vi "PH_SHS_Analysis_Calibrator.panel.vi"(0 "object ref":refnum<vi>, 5 "error in (no error)":errorcluster) -> (19 "error out":errorcluster)   [LabVIEW 2014, in "PH_SHS_Analysis_Calibrator.lvlib"]
doc: "The voltage measured by a device on high potential is represented by a frequency given out by a Beckhoff Klemme. This VI transforms it back into a voltage which wich is written to a memory tag. This value is indicated. In case of no connection (not mounted or bad tag value) or internal problems \"99999\" apears.\n\n\"Exit\" closes the GUI while \"Delete Instance\" additionally destroys the Instance.\n\n\n\nLicense Agreement for this software:\n\nCopyright (C)\nGesellschaft für Schwerionenforschung, GSI\nPlanckstr. 1\n64291 Darmstadt\nGermany\n\nContact: D.Beck@gsi.de \n\nThis program is free software; you can redistribute it and/or modify it under the terms of the GNU General Public License as published by the Free Software Foundation; either version 2 of the license, or (at your option) any later version.\n\nThis program is distributed in the hope that it will be useful, but WITHOUT ANYW ARRANTY; without even the implied warranty of MERCHANTABILITY or FITNESS FOR A PARTICULAR PURPOSE. See the GNU General License for more details (http://www.gnu.org).\n\nGesellschaft für Schwerionenforschung, GSI\nPlanckstr. 1, 64291 Darmstadt, Germany\nFor all questions and ideas contact: M.Richter@gsi.de, H.Brand@gsi.de or D.Beck@gsi.de.\nLast update: 18-DEC-2002"
uses:
  PH_SHS_Analysis_Calibrator.lvlib
  PH_Img_BaseClass/PH_Img_BaseClass.Palette.ctl
  PH_Img_BaseClass/PH_Img_BaseClass.GUI Refs.ctl
  PH_Common/PH_Common.lvlib
  PH_Img_BaseClass/PH_Img_BaseClass.lvlib
  CSCore/CSSystem/CSSystemLib/CSSystemLib.lvlib
  PH_Class/PH_Class.lvlib
panel:
  in  "Timeout Set":i32 caption="ms"
  in  "Palette":T1 items=["Grey", "Binary", "Gradient", "Rainbow", "Temperature"]
  out "Timeout":u32(colorbox)=16860
  out "Enough Images?":bool
  in  "Method":enum16{"automatic", "manual"}(ring)
  in  "MLA Pitch":dbl=200.0 caption="µm"
  in  "Pixel Size":dbl=6.7 caption="µm"
  out "Image":T2(plugin-control)
  out "Dialog":string
  in  "Repeat":bool
  in  "Skip":bool
  in  "Cancel":bool
  in  "OK":bool
  in  "Available Cams":u16(ring)
  in  "Delete":bool
  # "PCS"
  # "3.40"
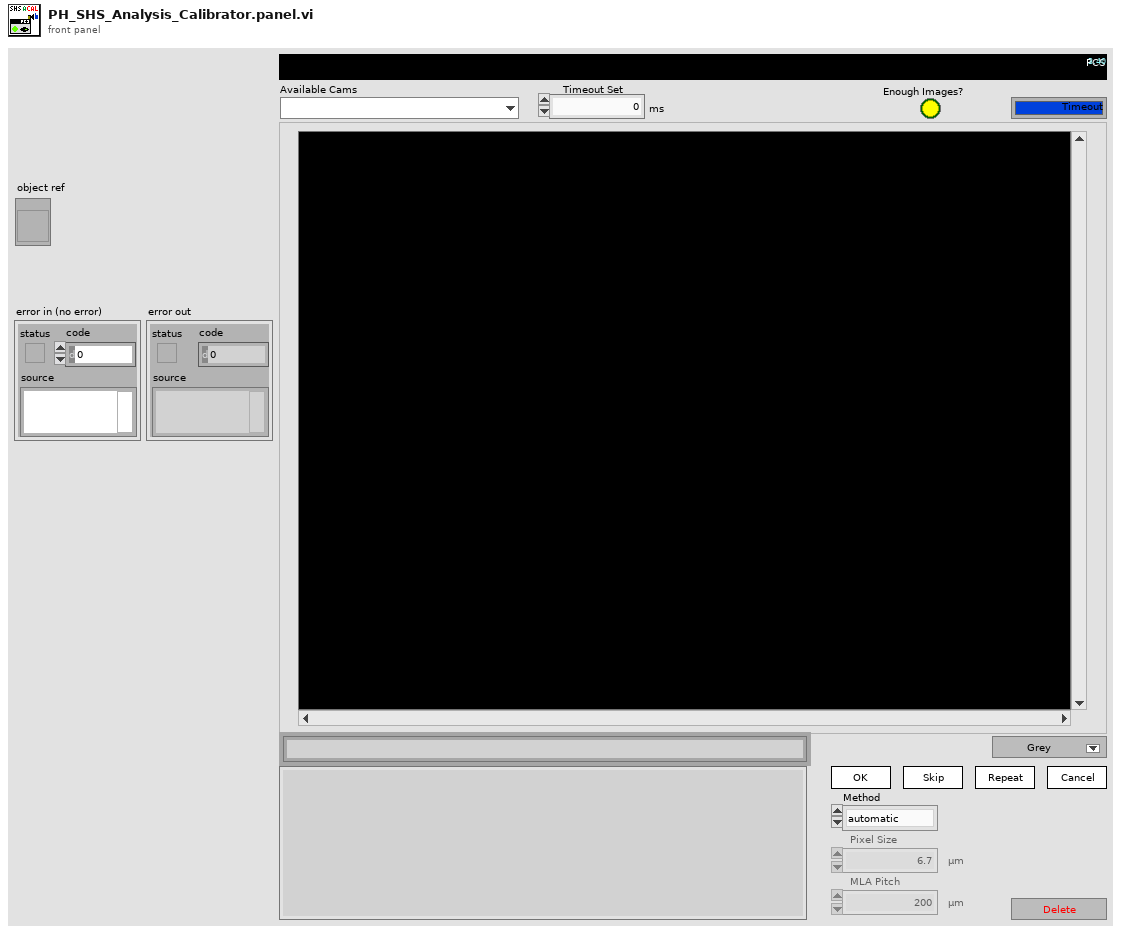
[diagram p1: front panel]
types:
  T1 = typedef "PH_Img_BaseClass.lvlib/PH_Img_BaseClass.Palette.ctl" = i32
  T2 = typedef "IMAQ Image.ctl" = refnum<image>
  T3 = typedef "PH_Img_BaseClass.lvlib/PH_Img_BaseClass.GUI Refs.ctl" = cluster{"Timeout":refnum<vi>, "Image":refnum<vi>, "Palette":refnum<vi>, "Timeout Set":refnum<vi>}
  T4 = enum8{"Enabled", "Disabled", "Disabled and Grayed Out"}
  T5 = typedef "PH_SHS_Analysis_Calibrator.lvlib/PH_SHS_Analysis_Calibrator.i attribute.ctl" = cluster{"GUI Refs":cluster{"Available Cams":refnum<vi>, "OK":refnum<vi>, "Skip":refnum<vi>, "Repeat":refnum<vi>, "Cancel":refnum<vi>, "Dialog":refnum<vi>, "Enough Images?":refnum<vi>}, "Cam instances":string[], "Status":cluster{"#":i32, "Data calculated":bool, "Wanted #":i32}, "IMAQ Image Array":T2[], "Pixel Size [µm]":dbl, "MLA Pitch [µm]":dbl, "Method":enum16{"automatic", "manual"}, "Enough Images?":bool, "SHS Reference Result":T6, "Calculation Error":errorcluster}
  T6 = typedef "SHS_Common.lvlib/SHSReference.ctl" = cluster{"Reference":T7[][], "Lens Array Pitch [px]":dbl}
  T7 = typedef "SHS_Common.lvlib/ReferencePoint.ctl" = cluster{"Rect":T8, "Point":T9}
  T8 = typedef "SHS_Common.lvlib/Rectangle.ctl" = cluster{"Left":i32, "Top":i32, "Right":i32, "Bottom":i32}
  T9 = typedef "SHS_Common.lvlib/Point.ctl" = cluster{"x":dbl, "y":dbl, "valid?":bool, "weight":dbl}
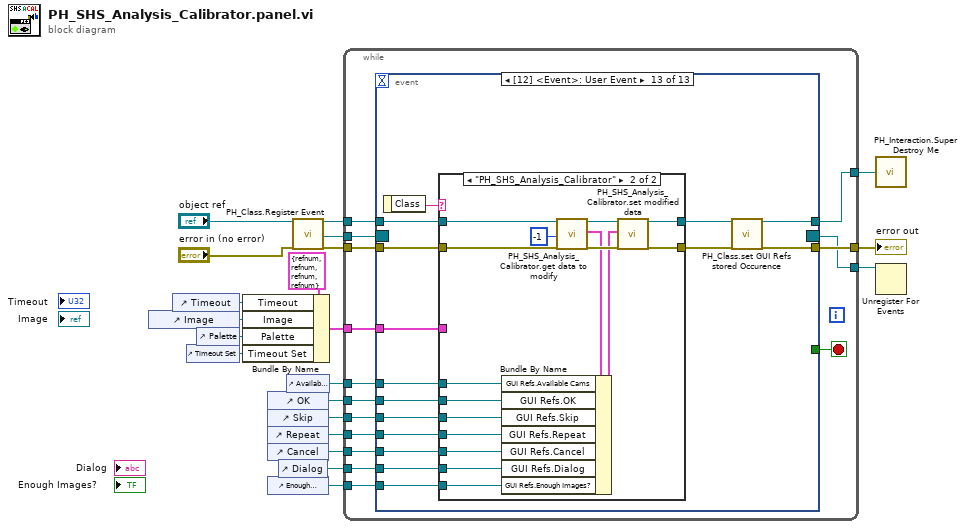
[diagram p0: block diagram]
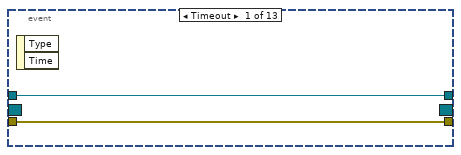
[diagram p2: hidden frame]
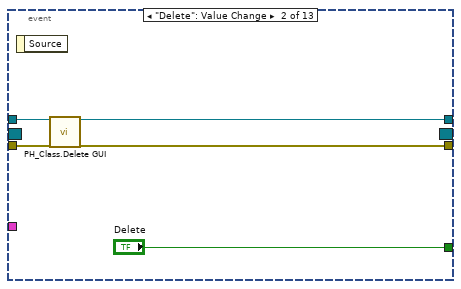
[diagram p3: hidden frame]
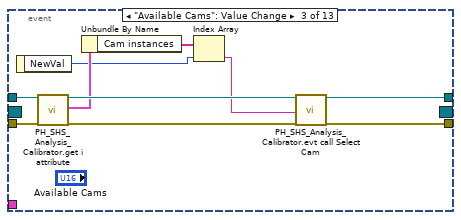
[diagram p4: hidden frame]
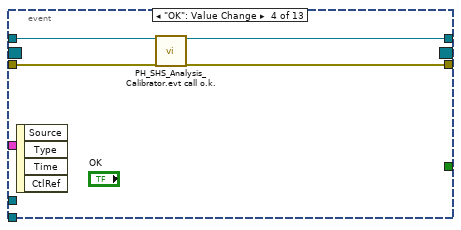
[diagram p5: hidden frame]
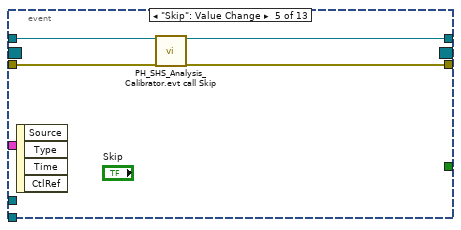
[diagram p6: hidden frame]
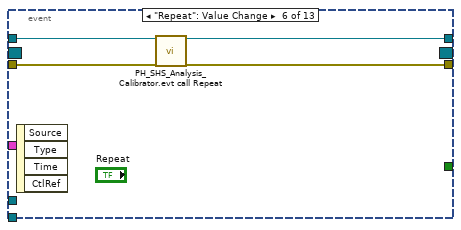
[diagram p7: hidden frame]
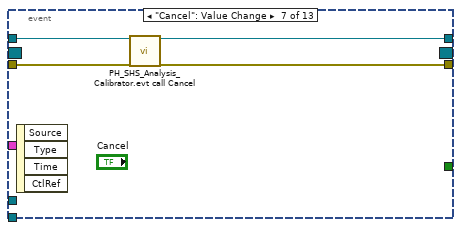
[diagram p8: hidden frame]
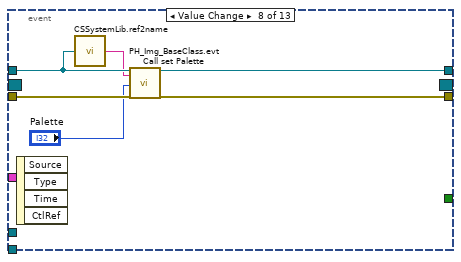
[diagram p9: hidden frame]
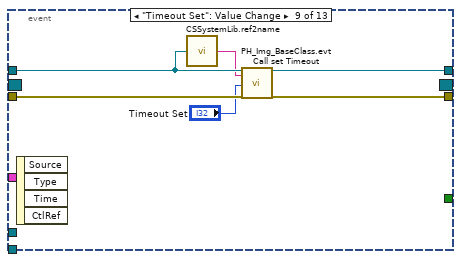
[diagram p10: hidden frame]
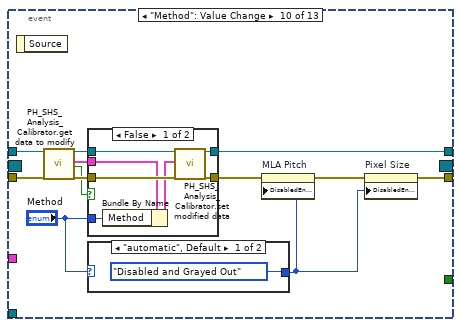
[diagram p11: hidden frame]
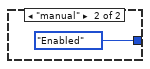
[diagram p12: hidden frame]
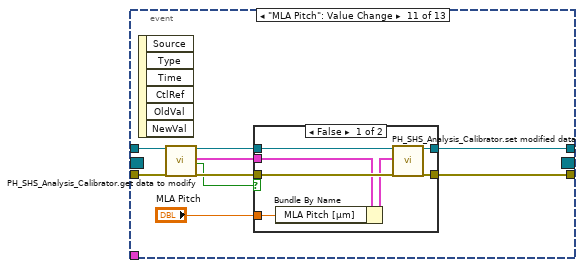
[diagram p14: hidden frame]
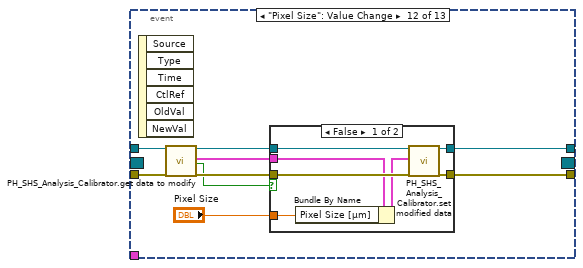
[diagram p16: hidden frame]
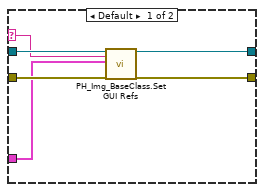
[diagram p18: hidden frame]
diagram:
  n1 = control-ref of="Image"() -> (w18:refnum<vi>)
  n2 = control-ref of="Timeout"() -> (w17:refnum<vi>)
  n3 = control-ref of="Timeout Set"() -> (w15:refnum<vi>)
  n4 = control-ref of="Palette"() -> (w16:refnum<vi>)
  n5 = Bundle By Name(cluster=T3 {"Timeout"=refnum, "Image"=refnum, "Palette"=refnum, "Timeout Set"=refnum} ("GUI Refs"), "Timeout"=w17, "Image"=w18, "Palette"=w16, "Timeout Set"=w15) -> (w3:T3)
  n6 = control-ref of="OK"() -> (w9:refnum<vi>)
  n7 = control-ref of="Skip"() -> (w8:refnum<vi>)
  n8 = control-ref of="Repeat"() -> (w7:refnum<vi>)
  n9 = control-ref of="Cancel"() -> (w6:refnum<vi>)
  n10 = control-ref of="Enough Images?"() -> (w4:refnum<vi>)
  n11 = control-ref of="Dialog"() -> (w5:refnum<vi>)
  n12 = control-ref of="Available Cams"() -> (w10:refnum<vi>)
  n13 = call "PH_Class.Register Event.vi"("i ref in"="object ref", "error in (no error)"="error in (no error)") -> ("i ref out"=w14:refnum<vi>, "Event Registration Refnum"=w12:refnum<event-registration>, "error out"=w13:errorcluster)  [unwired: 15 in]
  n14 = while {
    tunnel: w14 -> [w33]
    tunnel: [w32] -> w21
    tunnel: w13 -> [w35]
    tunnel: [w34] -> w20
    tunnel: w12 -> [w31]
    tunnel: [w30] -> w11
    tunnel: w10 -> [w29]
    tunnel: w9 -> [w28]
    tunnel: w8 -> [w27]
    tunnel: w7 -> [w26]
    tunnel: w6 -> [w25]
    tunnel: w5 -> [w24]
    tunnel: w4 -> [w23]
    tunnel: w3 -> [w22]
    stop <- w36 stop-if-true
    n15 = event shown="[12] <Event>: User Event" {
      selector: w31 -> [_ _ _ _ _ _ _ _ _ _ _ _ _]
      dyn-events: [_ _ _ _ _ _ _ _ _ _ _ _ _] -> w30
      timeout: _ -> [_ _ _ _ _ _ _ _ _ _ _ _ _]
      tunnel: [_ "Delete" _ _ _ _ _ _ _ _ _ _ _] -> w36
      tunnel: w33 -> [w37 w42 w50 w57 w61 w65 w68 w71 w78 w93 w113 w131 w153]
      tunnel: w35 -> [w38 w41 w52 w56 w60 w64 w69 w75 w81 w92 w112 w130 w151]
      tunnel: [w38 w39 w53 w55 w59 w63 w67 w74 w80 w84 w106 w124 w154] -> w34
      tunnel: [w37 w40 w44 w54 w58 w62 w66 w73 w79 w89 w109 w127 w155] -> w32
      tunnel: w29 -> [_ _ _ _ _ _ _ _ _ _ _ _ w148]
      tunnel: w28 -> [_ _ _ _ _ _ _ _ _ _ _ _ w147]
      tunnel: w27 -> [_ _ _ _ _ _ _ _ _ _ _ _ w146]
      tunnel: w26 -> [_ _ _ _ _ _ _ _ _ _ _ _ w145]
      tunnel: w25 -> [_ _ _ _ _ _ _ _ _ _ _ _ w144]
      tunnel: w24 -> [_ _ _ _ _ _ _ _ _ _ _ _ w143]
      tunnel: w23 -> [_ _ _ _ _ _ _ _ _ _ _ _ w142]
      tunnel: w22 -> [_ _ _ _ _ _ _ _ _ _ _ _ w141]
      event Timeout {
        n16 = event-data() -> ()  [unwired: 1 in, 2 out]
      }
      event "Delete": Value Change {
        n17 = event-data() -> ()  [unwired: 1 in, 1 out]
        n18 = call "PH_Class.Delete GUI.vi"("VI in"=w42, "error in (no error)"=w41) -> ("VI out"=w40:refnum<vi>, "error out"=w39:errorcluster)  [unwired: 16 in]
      }
      event "Available Cams": Value Change {
        n19 = event-data() -> ("NewVal"=w46:u16)  [unwired: 1 in]
        n20 = call "PH_SHS_Analysis_Calibrator.get i attribute.vi"("i ref in"=w50, "error in (no error)"=w52) -> ("i ref out"=w49:refnum<vi>, "i attribute"=w48:T5, "error out"=w51:errorcluster)  [unwired: 15 in]
        n21 = Unbundle By Name(w48) -> ("Cam instances"=w47:string[])
        n22 = Index Array(array=w47, index=w46) -> (element=w45:string)
        n23 = call "PH_SHS_Analysis_Calibrator.evt call Select Cam.vi"("i ref in"=w49, "Cam"=w45, "error in"=w51) -> ("i ref out"=w44:refnum<vi>, "error out"=w53:errorcluster)  [unwired: 15 in]
      }
      event "OK": Value Change {
        n24 = event-data() -> ()  [unwired: 1 in, 4 out]
        n25 = call "PH_SHS_Analysis_Calibrator.evt call o.k..vi"("i ref in"=w57, "error in"=w56) -> ("i ref out"=w54:refnum<vi>, "error out"=w55:errorcluster)  [unwired: 16 in]
      }
      event "Skip": Value Change {
        n26 = event-data() -> ()  [unwired: 1 in, 4 out]
        n27 = call "PH_SHS_Analysis_Calibrator.evt call Skip.vi"("i ref in"=w61, "error in"=w60) -> ("i ref out"=w58:refnum<vi>, "error out"=w59:errorcluster)  [unwired: 16 in]
      }
      event "Repeat": Value Change {
        n28 = event-data() -> ()  [unwired: 1 in, 4 out]
        n29 = call "PH_SHS_Analysis_Calibrator.evt call Repeat.vi"("i ref in"=w65, "error in"=w64) -> ("i ref out"=w62:refnum<vi>, "error out"=w63:errorcluster)  [unwired: 16 in]
      }
      event "Cancel": Value Change {
        n30 = event-data() -> ()  [unwired: 1 in, 4 out]
        n31 = call "PH_SHS_Analysis_Calibrator.evt call Cancel.vi"("i ref in"=w68, "error in"=w69) -> ("i ref out"=w66:refnum<vi>, "error out"=w67:errorcluster)  [unwired: 16 in]
      }
      event Value Change {
        n32 = event-data() -> ()  [unwired: 1 in, 4 out]
        n33 = call "CSSystemLib.ref2name.vi"("obj refnum"=w71) -> ("name"=w70:string)
        n34 = call "PH_Img_BaseClass.evt Call set Palette.vi"("i ref in"=w71, "Instance"=w70, "Palette"="Palette", "error in (no error)"=w75) -> ("i ref out"=w73:refnum<vi>, "error out"=w74:errorcluster)  [unwired: 14 in]
      }
      event "Timeout Set": Value Change {
        n35 = event-data() -> ()  [unwired: 1 in, 4 out]
        n36 = call "CSSystemLib.ref2name.vi"("obj refnum"=w78) -> ("name"=w77:string)
        n37 = call "PH_Img_BaseClass.evt Call set Timeout.vi"("i ref in"=w78, "Instance"=w77, "Timeout [ms]"="Timeout Set", "error in (no error)"=w81) -> ("i ref out"=w79:refnum<vi>, "error out"=w80:errorcluster)  [unwired: 14 in]
      }
      event "Method": Value Change {
        n38 = event-data() -> ()  [unwired: 1 in, 1 out]
        n39 = call "PH_SHS_Analysis_Calibrator.get data to modify.vi"("i ref in"=w93, "error in (no error)"=w92) -> ("i ref out"=w90:refnum<vi>, "i attribute"=w87:T5, "timed out"=w88:bool, "error out"=w91:errorcluster)  [unwired: 14 in]
        n40 = case shown="False" w88 {
          tunnel: w91 -> [w102 w103]
          tunnel: w90 -> [w101 w104]
          tunnel: [w100 w104] -> w89
          tunnel: [w99 w103] -> w86
          tunnel: w87 -> [w98 _]
          tunnel: "Method" -> [w96 _]
          frame False {
            n41 = Bundle By Name(cluster=w98, "Method"=w96) -> (w97:T5)
            n42 = call "PH_SHS_Analysis_Calibrator.set modified data.vi"("i ref in"=w101, "i attribute"=w97, "error in (no error)"=w102) -> ("i ref out"=w100:refnum<vi>, "error out"=w99:errorcluster)  [unwired: 15 in]
          }
          frame True {
          }
        }
        n43 = case shown="\"automatic\", Default" "Method" {
          tunnel: [T4."Disabled and Grayed Out" ("Disabled") T4."Enabled" ("Disabled")] -> w82
          frame "automatic", Default {
          }
          frame "manual" {
          }
        }
        n44 = property on="MLA Pitch" class="DigNum (strict)"(error in=w86, "DisabledEnum"=w82) -> (error out=w85:errorcluster)  [unwired: 1 in, 1 out]
        n45 = property on="Pixel Size" class="DigNum (strict)"(error in=w85, "DisabledEnum"=w82) -> (error out=w84:errorcluster)  [unwired: 1 in, 1 out]
      }
      event "MLA Pitch": Value Change {
        n46 = event-data() -> ()  [unwired: 1 in, 6 out]
        n47 = call "PH_SHS_Analysis_Calibrator.get data to modify.vi"("i ref in"=w113, "error in (no error)"=w112) -> ("i ref out"=w110:refnum<vi>, "i attribute"=w107:T5, "timed out"=w108:bool, "error out"=w111:errorcluster)  [unwired: 14 in]
        n48 = case shown="False" w108 {
          tunnel: w111 -> [w120 w121]
          tunnel: w110 -> [w119 w122]
          tunnel: [w118 w122] -> w109
          tunnel: [w117 w121] -> w106
          tunnel: w107 -> [w116 _]
          tunnel: "MLA Pitch" -> [w114 _]
          frame False {
            n49 = Bundle By Name(cluster=w116, "MLA Pitch [µm]"=w114) -> (w115:T5)
            n50 = call "PH_SHS_Analysis_Calibrator.set modified data.vi"("i ref in"=w119, "i attribute"=w115, "error in (no error)"=w120) -> ("i ref out"=w118:refnum<vi>, "error out"=w117:errorcluster)  [unwired: 15 in]
          }
          frame True {
          }
        }
      }
      event "Pixel Size": Value Change {
        n51 = event-data() -> ()  [unwired: 1 in, 6 out]
        n52 = call "PH_SHS_Analysis_Calibrator.get data to modify.vi"("i ref in"=w131, "error in (no error)"=w130) -> ("i ref out"=w128:refnum<vi>, "i attribute"=w125:T5, "timed out"=w126:bool, "error out"=w129:errorcluster)  [unwired: 14 in]
        n53 = case shown="False" w126 {
          tunnel: w129 -> [w138 w139]
          tunnel: w128 -> [w137 w140]
          tunnel: [w136 w140] -> w127
          tunnel: [w135 w139] -> w124
          tunnel: w125 -> [w134 _]
          tunnel: "Pixel Size" -> [w132 _]
          frame False {
            n54 = Bundle By Name(cluster=w134, "Pixel Size [µm]"=w132) -> (w133:T5)
            n55 = call "PH_SHS_Analysis_Calibrator.set modified data.vi"("i ref in"=w137, "i attribute"=w133, "error in (no error)"=w138) -> ("i ref out"=w136:refnum<vi>, "error out"=w135:errorcluster)  [unwired: 15 in]
          }
          frame True {
          }
        }
      }
      event User Event {
        n56 = event-data() -> ("Class"=w149:string)  [unwired: 1 in]
        n57 = case shown="\"PH_SHS_Analysis_Calibrator\"" w149 {
          selector: w149 -> [w156 _]
          tunnel: w153 -> [w161 w172]
          tunnel: [w159 w171] -> w152
          tunnel: w151 -> [w160 w170]
          tunnel: [w158 w169] -> w150
          tunnel: w148 -> [_ w168]
          tunnel: w147 -> [_ w167]
          tunnel: w146 -> [_ w166]
          tunnel: w145 -> [_ w165]
          tunnel: w144 -> [_ w164]
          tunnel: w143 -> [_ w163]
          tunnel: w142 -> [_ w162]
          tunnel: w141 -> [w157 _]
          frame Default {
            n58 = call "PH_Img_BaseClass.Set GUI Refs.vi"("i ref in"=w161, "Class"=w156, "GUI Refs"=w157, "error in (no error)"=w160) -> ("i ref out"=w159:refnum<vi>, "error out"=w158:errorcluster)  [unwired: 14 in]
          }
          frame "PH_SHS_Analysis_Calibrator" {
            n59 = call "PH_SHS_Analysis_Calibrator.get data to modify.vi"("i ref in"=w172, "ms timeout (10000)"=-1, "error in (no error)"=w170) -> ("i ref out"=w177:refnum<vi>, "i attribute"=w174:T5, "error out"=w176:errorcluster)  [unwired: 13 in, 1 out]
            n60 = Bundle By Name(cluster=w174, "GUI Refs.Available Cams"=w168, "GUI Refs.OK"=w167, "GUI Refs.Skip"=w166, "GUI Refs.Repeat"=w165, "GUI Refs.Cancel"=w164, "GUI Refs.Dialog"=w163, "GUI Refs.Enough Images?"=w162) -> (w173:T5)
            n61 = call "PH_SHS_Analysis_Calibrator.set modified data.vi"("i ref in"=w177, "i attribute"=w173, "error in (no error)"=w176) -> ("i ref out"=w171:refnum<vi>, "error out"=w169:errorcluster)  [unwired: 15 in]
          }
        }
        n62 = call "PH_Class.set GUI Refs stored Occurence.vi"("i ref in"=w152, "error in (no error)"=w150) -> ("i ref out"=w155:refnum<vi>, "error out"=w154:errorcluster)  [unwired: 16 in]
      }
    }
  }
  "error out" <- w20
  n63 = call "PH_Interaction.Super Destroy Me.vi"("i ref out"=w21) -> ()
  n64 = Unregister For Events(event registration refnum=w11) -> ()  [unwired: 1 in, 1 out]
